vi "Angle_3.vi"() -> ()   [LabVIEW 2020]
uses:
  Support/Controls/Cmd_Mouse Popup.ctl
  Support/Controls/Clst_Initialize Input.ctl
  Support/Controls/Clst_Result inspec.ctl
  Support/Controls/Cmd_Var Data IO.ctl
  Variables/Global_Cal Info.vi
panel:
  in  "반지름":string="150" caption="투영면 반지름 (mm)"
  out "최소범위":string
  in  "표시방식":string(combo)
  out "단위":string
  out "최대범위":string
  in  "Spec 변경":bool
  in  "Random":bool
  out "Resolution":string[][](table) caption="Spec"
  out "Spec":string[][](table)
  out "제목":string
  out "에러 출력":errorcluster
  out "Condition":string[][](table) caption="2. 직선성 시험"
  in  "최소눈금":string(combo)
  in  "Measured":string[][](table) caption="투영면의 회전 각도 측정오차"
  out "Load?":bool
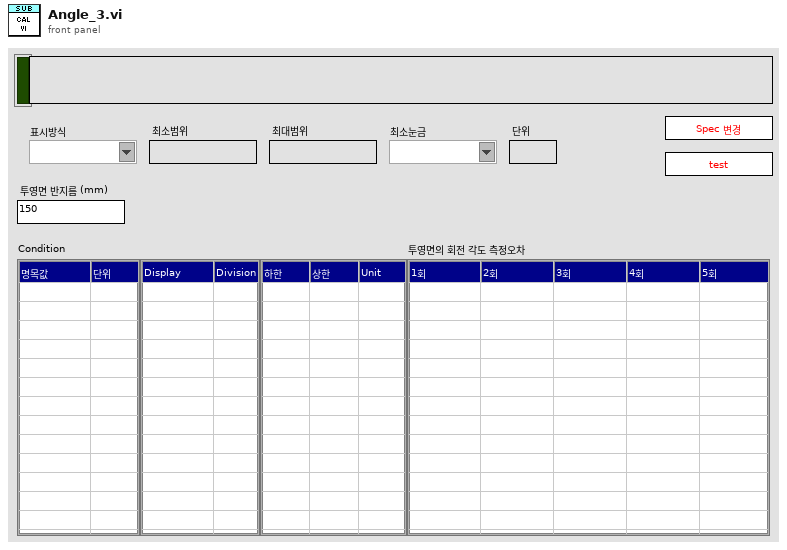
[diagram p1: front panel]
types:
  T1 = typedef "Cmd_Mouse Popup.ctl" = enum16{"활성화", "메뉴선택"}
  T2 = cluster{"Shift":bool, "Ctrl":bool, "Alt":bool, "Cmd":bool, "Opt":bool}
  T3 = typedef "Clst_Initialize Input.ctl" = cluster{"Initialize 1":cluster{"Condition":refnum<vi>[], "Spec":refnum<vi>[], "Measured":refnum<vi>[], "Resolution":refnum<vi>[], "Func_ext":string, "제목":refnum<vi>, "Measured_ADJ":refnum<vi>[]}, "Initialize 2":cluster{"문자열":refnum<vi>[], "콤보박스":refnum<vi>[], "링":refnum<vi>[], "열거형":refnum<vi>[], "테이블":refnum<vi>[], "여러열":refnum<vi>[], "디지털(DBL)":refnum<vi>[], "3D string":refnum<vi>[], "ctrl":refnum<vi>[], "boolean":refnum<vi>[]}}
  T4 = typedef "Clst_Result inspec.ctl" = cluster{"분해능":string, "문자열 1":string, "문자열 2":string, "숫자형 1":i32, "숫자형 2":i32, "숫자형 3":dbl, "문자배열 1D":string[], "문자배열 2D":string[][], "문자배열 3D":string[][][], "문자배열 4D":string[][][][], "불리언 1D":bool[]}
  T5 = typedef "Cmd_Var Data IO.ctl" = enum16{"Condition", "Condition Default", "Condition_Temp", "Resolution", "Resolution Default", "Resolution Old", "Spec", "Spec Default", "Spec Old", "Spec Temp", "Result", "Result2", "Result3", "Result_Temp", "Result_ADJ", "Result_ADJ2", "STD1", "STD2", "STD3", "STD4", "STD5", "STD Temp", "CMC", "CMC Default"}
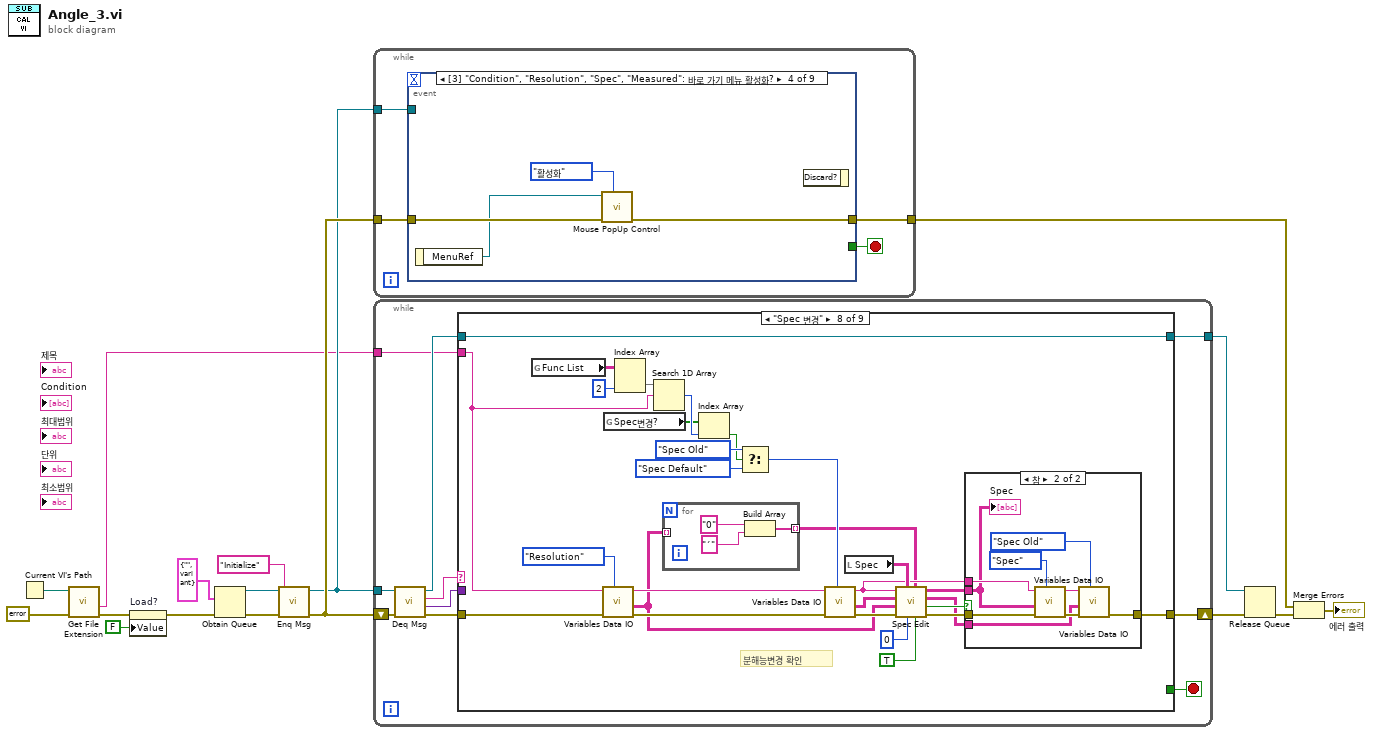
[diagram p0: block diagram]
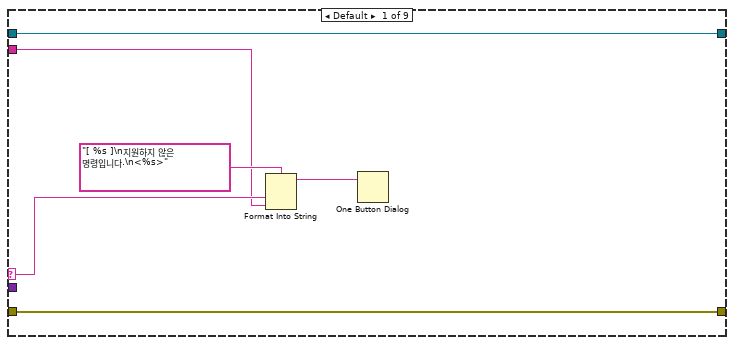
[diagram p2: hidden frame]
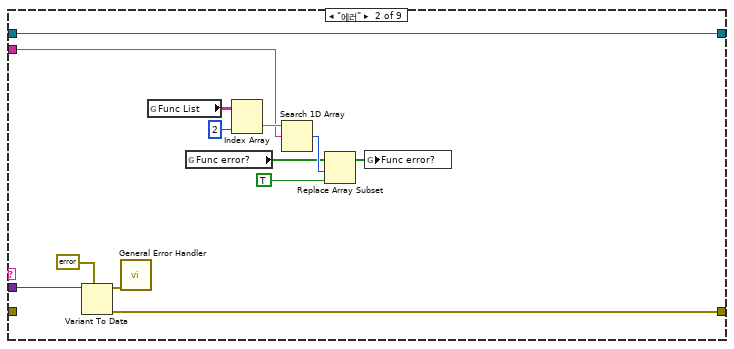
[diagram p3: hidden frame]
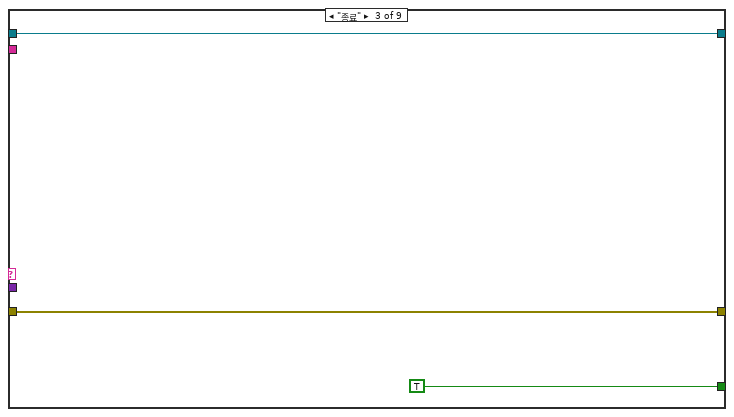
[diagram p4: hidden frame]
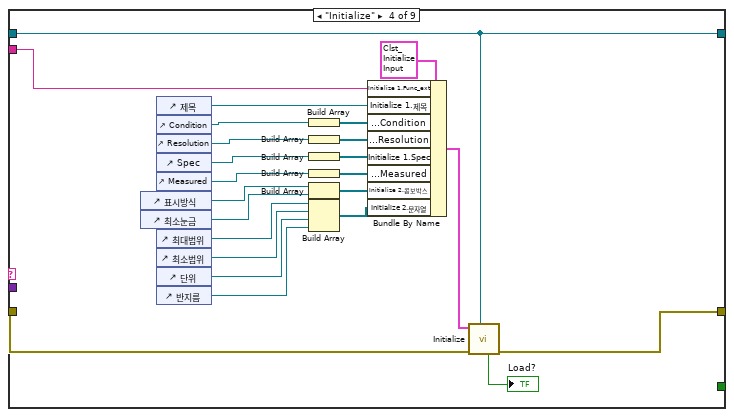
[diagram p5: hidden frame]
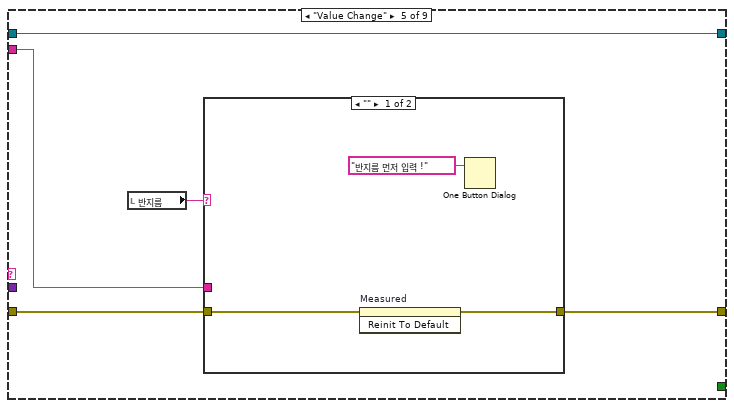
[diagram p6: hidden frame]
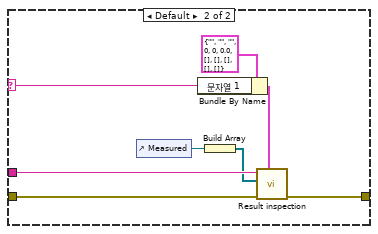
[diagram p7: hidden frame]
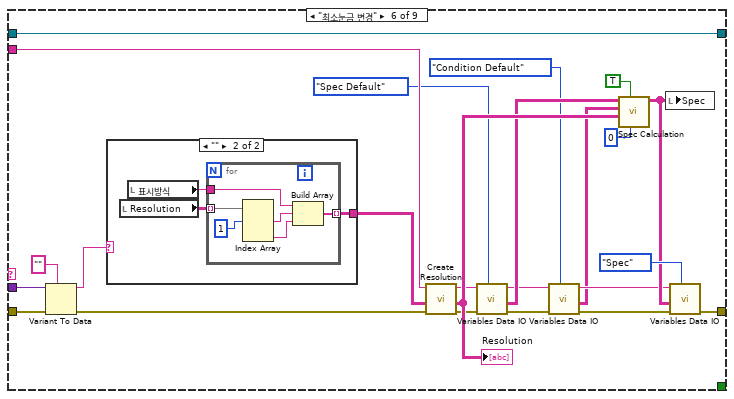
[diagram p8: hidden frame]
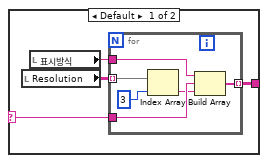
[diagram p9: hidden frame]
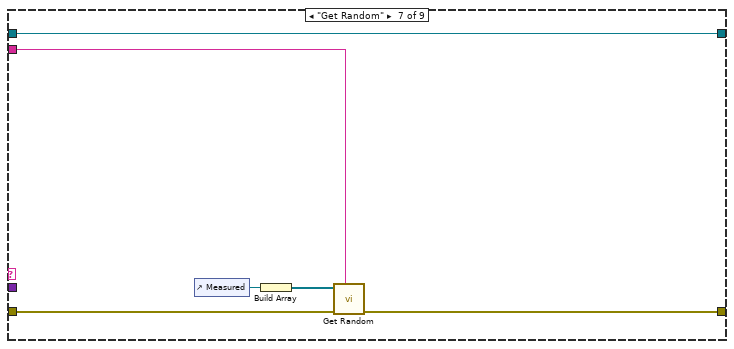
[diagram p10: hidden frame]
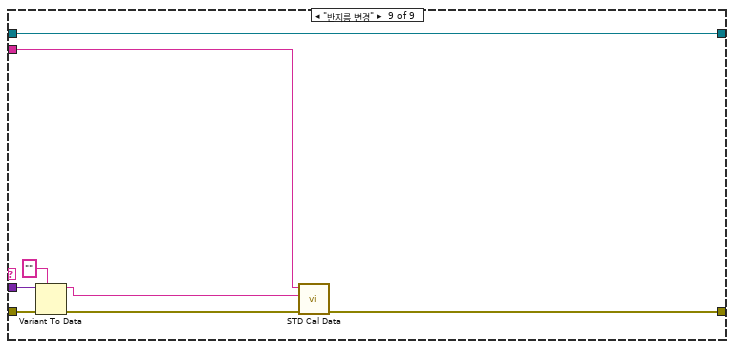
[diagram p12: hidden frame]
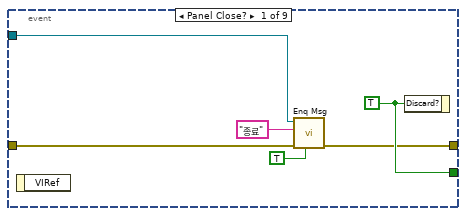
[diagram p13: hidden frame]
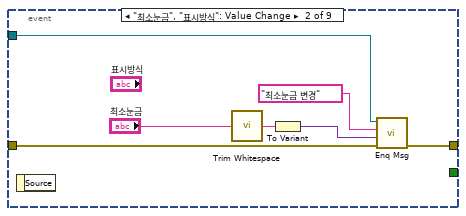
[diagram p14: hidden frame]
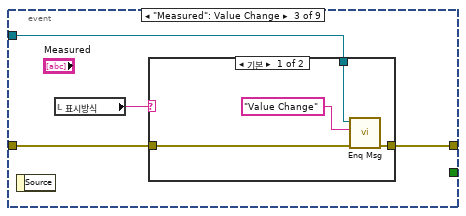
[diagram p15: hidden frame]
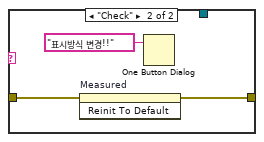
[diagram p16: hidden frame]
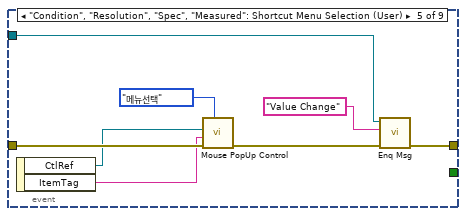
[diagram p17: hidden frame]
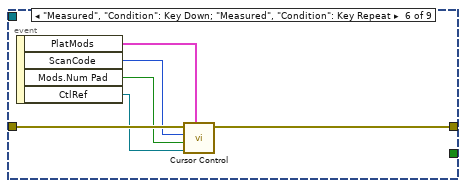
[diagram p18: hidden frame]
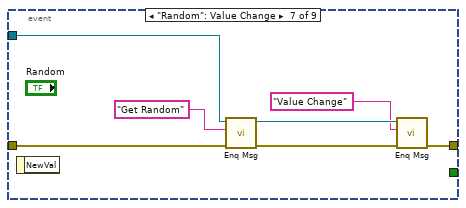
[diagram p19: hidden frame]
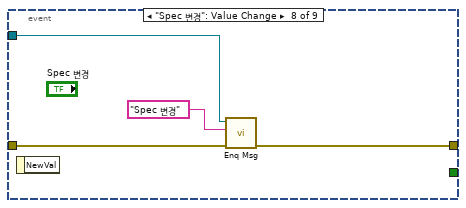
[diagram p20: hidden frame]
diagram:
  n1 = Current VI's Path() -> (path=w5:path)
  n2 = call <vilib>:"Get File Extension.vi"("error in (no error)"=errorcluster {"status"=FALSE, "code"=0, "source"=""} ("에러 상수"), "file"=w5) -> ("error out"=w3:errorcluster, "filename without extension"=w4:string)  [unwired: 5 in, 3 out]
  n3 = property on="Load?" class="Bool (엄격한)"(error in=w3, "Value"=FALSE ("Load?")) -> (error out=w2:errorcluster)  [unwired: 1 in, 1 out]
  n4 = Obtain Queue(element data type=cluster{"메세지":string, "값":variant} {"메세지"="", "값"=variant} ("Message Cluster"), error in (no error)=w2) -> (queue out=w14:refnum<queue>, error out=w16:errorcluster)  [unwired: 3 in, 1 out]
  n5 = call "Enq Msg.vi"("에러 입력(에러 없음)"=w16, "메세지"="Initialize", "큐 입력"=w14) -> ("에러 출력"=w15:errorcluster, "큐 출력"=w12:refnum<queue>)  [unwired: 7 in]
  n6 = while {
    tunnel: w15 -> [w19]
    tunnel: w12 -> [w20]
    tunnel: [w18] -> w9
    stop <- w21 stop-if-true
    n7 = event shown="[3] \"Condition\", \"Resolution\", \"Spec\", \"Measured\": 바로 가기 메뉴 활성화?" {
      selector: _ -> [_ _ _ _ _ _ _ _ _]
      dyn-events: _ -> [_ _ _ _ _ _ _ _ _]
      timeout: _ -> [_ _ _ _ _ _ _ _ _]
      tunnel: [w27 _ _ _ _ _ _ _ _] -> w21
      tunnel: w20 -> [w25 w33 w38 _ w50 _ w68 w72 w75]
      tunnel: w19 -> [w26 w34 w36 w49 w57 w63 w69 w73 w79]
      tunnel: [w23 w32 w37 w48 w51 w62 w64 w71 w78] -> w18
      event Panel Close? {
        w27 = TRUE ("버림?")
        n8 = event-data() -> ()  [unwired: 1 in, 1 out]
        n9 = call "Enq Msg.vi"("우선순위 메시지?"=TRUE, "에러 입력(에러 없음)"=w26, "메세지"="종료", "큐 입력"=w25) -> ("에러 출력"=w23:errorcluster)  [unwired: 6 in, 1 out]
        n10 = event-data("Discard?"=w27) -> ()  [unwired: 1 in, 1 out]
      }
      event "최소눈금", "표시방식": Value Change {
        n11 = event-data() -> ()  [unwired: 1 in, 1 out]
        n12 = call <vilib>:"Trim Whitespace.vi"("string"="최소눈금") -> ("trimmed string"=w30:string)  [unwired: 1 in]
        n13 = To Variant(anything=w30) -> (Variant=w28:variant)
        n14 = call "Enq Msg.vi"("에러 입력(에러 없음)"=w34, "값"=w28, "메세지"="최소눈금 변경", "큐 입력"=w33) -> ("에러 출력"=w32:errorcluster)  [unwired: 6 in, 1 out]
      }
      event "Measured": Value Change {
        n15 = event-data() -> ()  [unwired: 1 in, 1 out]
        n16 = local read "표시방식"() -> (w35:string)
        n17 = case shown="기본" w35 {
          tunnel: w38 -> [w42 _]
          tunnel: [w41 w43] -> w37
          tunnel: w36 -> [w40 w44]
          frame Default {
            n18 = call "Enq Msg.vi"("에러 입력(에러 없음)"=w40, "메세지"="Value Change", "큐 입력"=w42) -> ("에러 출력"=w41:errorcluster)  [unwired: 7 in, 1 out]
          }
          frame "Check" {
            n19 = invoke on="Measured" class="Tbl (엄격한)" method="Reinit To Default"(error in=w44) -> (error out=w43:errorcluster)  [unwired: 2 in, 2 out]
            n20 = One Button Dialog(message="표시방식 변경!!" ("메시지")) -> ()  [unwired: 1 in, 1 out]
          }
        }
      }
      event "Condition", "Resolution", "Spec", "Measured": Shortcut Menu Activation? {
        n21 = event-data() -> ("MenuRef"=w47:refnum<k9>)  [unwired: 1 in]
        n22 = call "Mouse PopUp Control.vi"("type"=Cmd_Mouse_Popup."활성화", "error in"=w49, "메뉴 참조"=w47) -> ("error out"=w48:errorcluster)  [unwired: 8 in]
        n23 = event-data() -> ()  [unwired: 2 in, 1 out]
      }
      event "Condition", "Resolution", "Spec", "Measured": Shortcut Menu Selection (User) {
        n24 = event-data() -> ("CtlRef"=w55:refnum<vi>, "ItemTag"=w54:string)  [unwired: 1 in]
        n25 = call "Mouse PopUp Control.vi"("type"=Cmd_Mouse_Popup."메뉴선택", "error in"=w57, "아이템 태그"=w54, "Tbl 참조 번호"=w55) -> ("error out"=w52:errorcluster)  [unwired: 7 in]
        n26 = call "Enq Msg.vi"("에러 입력(에러 없음)"=w52, "메세지"="Value Change", "큐 입력"=w50) -> ("에러 출력"=w51:errorcluster)  [unwired: 7 in, 1 out]
      }
      event "Measured", "Condition": Key Down; "Measured", "Condition": Key Repeat {
        n27 = event-data() -> ("PlatMods"=w58:T2, "ScanCode"=w61:i16, "Mods.Num Pad"=w60:bool, "CtlRef"=w59:refnum<vi>)  [unwired: 1 in]
        n28 = call "Cursor Control.vi"("플랫폼 조합키"=w58, "참조"=w59, "Num Pad"=w60, "ScanCode"=w61, "error in"=w63) -> ("error out"=w62:errorcluster)  [unwired: 5 in, 1 out]
      }
      event "Random": Value Change {
        n29 = event-data() -> ()  [unwired: 1 in, 1 out]
        n30 = call "Enq Msg.vi"("에러 입력(에러 없음)"=w69, "메세지"="Get Random", "큐 입력"=w68) -> ("에러 출력"=w67:errorcluster, "큐 출력"=w66:refnum<queue>)  [unwired: 7 in]
        n31 = call "Enq Msg.vi"("에러 입력(에러 없음)"=w67, "메세지"="Value Change", "큐 입력"=w66) -> ("에러 출력"=w64:errorcluster)  [unwired: 7 in, 1 out]
      }
      event "Spec 변경": Value Change {
        n32 = event-data() -> ()  [unwired: 1 in, 1 out]
        n33 = call "Enq Msg.vi"("에러 입력(에러 없음)"=w73, "메세지"="Spec 변경", "큐 입력"=w72) -> ("에러 출력"=w71:errorcluster)  [unwired: 7 in, 1 out]
      }
      event "반지름": Value Change {
        n34 = event-data() -> ()  [unwired: 1 in, 2 out]
        n35 = To Variant(anything="반지름") -> (Variant=w76:variant)
        n36 = call "Enq Msg.vi"("에러 입력(에러 없음)"=w79, "값"=w76, "메세지"="반지름 변경", "큐 입력"=w75) -> ("에러 출력"=w78:errorcluster)  [unwired: 6 in, 1 out]
      }
    }
  }
  n37 = while {
    shift-right: [w90] -> w11
    shift-left: w15 -> [w89]
    tunnel: w12 -> [w87]
    tunnel: [w82] -> w10
    tunnel: w4 -> [w81]
    stop <- w83 stop-if-true
    n38 = call "Deq Msg.vi"("에러 입력(에러 없음)"=w89, "큐 입력"=w87) -> ("에러 출력"=w88:errorcluster, "값"=w84:variant, "메세지"=w86:string, "큐 출력"=w85:refnum<queue>)  [unwired: 6 in]
    n39 = case shown="\"Spec 변경\"" w86 {
      selector: w86 -> [w92 _ _ _ _ _ _ _ _]
      tunnel: w88 -> [w96 _ w112 w136 w138 w175 w197 w222 w249]
      tunnel: [w96 w106 w112 w116 w140 w168 w198 w225 w243] -> w90
      tunnel: w85 -> [w95 w105 w110 w121 w141 w176 w201 w229 w250]
      tunnel: w84 -> [_ w107 _ _ _ w174 _ _ w247]
      tunnel: [_ _ TRUE ("버림?") _ _ _ _ _ _] -> w83
      tunnel: [w95 w105 w110 w121 w141 w176 w201 w229 w250] -> w82
      tunnel: w81 -> [w91 w97 _ w122 w139 w172 w196 w208 w244]
      frame Default {
        n40 = Format Into String(format string="[ %s ]\n지원하지 않은 명령입니다.\n<%s>" ("메시지"), w92, w91) -> (resulting string=w93:string)  [unwired: 2 in, 1 out]
        n41 = One Button Dialog(message=w93) -> ()  [unwired: 1 in, 1 out]
      }
      frame "에러" {
        n42 = Variant To Data(type=errorcluster {"status"=FALSE, "code"=0, "source"=""} ("에러 출력"), Variant=w107) -> (data=w109:errorcluster, error out=w106:errorcluster)  [unwired: 1 in]
        n43 = call <vilib>:"General Error Handler.vi"("error in (no error)"=w109) -> ()  [unwired: 10 in, 5 out]
        n44 = global read "Global_Cal Info.vi" "Func List"() -> (w99:string[][])
        n45 = global read "Global_Cal Info.vi" "Func error?"() -> (w102:bool[])
        n46 = Index Array(array=w99, index (col)=2 ("비활성화된 인덱스 (열)")) -> (element=w100:string[])  [unwired: 1 in]
        n47 = Search 1D Array(1D array=w100, element=w97) -> (index of element=w103:i32)  [unwired: 1 in]
        n48 = Replace Array Subset(array=w102, new element=TRUE ("새 원소/부분배열"), index=w103) -> (w104:bool[])
        n49 = global write "Global_Cal Info.vi" "Func error?"(w104) -> ()
      }
      frame "종료" {
      }
      frame "Initialize" {
        n50 = control-ref of="표시방식"() -> (w120:refnum<vi>)
        n51 = control-ref of="최소눈금"() -> (w129:refnum<vi>)
        n52 = control-ref of="제목"() -> (w127:refnum<vi>)
        n53 = control-ref of="Condition"() -> (w133:refnum<vi>)
        n54 = control-ref of="Resolution"() -> (w123:refnum<vi>)
        n55 = control-ref of="Spec"() -> (w126:refnum<vi>)
        n56 = control-ref of="Measured"() -> (w130:refnum<vi>)
        n57 = control-ref of="최대범위"() -> (w115:refnum<vi>)
        n58 = control-ref of="최소범위"() -> (w117:refnum<vi>)
        n59 = control-ref of="단위"() -> (w119:refnum<vi>)
        n60 = control-ref of="반지름"() -> (w113:refnum<vi>)
        n61 = Build Array(w133) -> (w132:refnum<vi>[])
        n62 = Build Array(w123) -> (w124:refnum<vi>[])
        n63 = Build Array(w126) -> (w125:refnum<vi>[])
        n64 = Build Array(w130) -> (w131:refnum<vi>[])
        n65 = Build Array(w120, w129) -> (w128:refnum<vi>[])
        n66 = Build Array(w115, w117, w119, w113) -> (w118:refnum<vi>[])
        n67 = Bundle By Name(cluster=T3 {"Initialize 1"={"Condition"=[], "Spec"=[], "Measured"=[], "Resolution"=[], "Func_ext"="", "제목"=refnum, "Measured_ADJ"=[]}, "Initialize 2"={"문자열"=[], "콤보박스"=[], "링"=[], "열거형"=[], "테이블"=[], "여러열"=[], "디지털(DBL)"=[], "3D string"=[], "ctrl"=[], "boolean"=[]}} ("입력 클러스터"), "Initialize 1.Func_ext"=w122, "Initialize 1.제목"=w127, "Initialize 1.Condition"=w132, "Initialize 1.Resolution"=w124, "Initialize 1.Spec"=w125, "Initialize 1.Measured"=w131, "Initialize 2.콤보박스"=w128, "Initialize 2.문자열"=w118) -> (w134:T3)
        n68 = call "Initialize.vi"("큐 입력"=w121, "error in"=w136, "입력 클러스터"=w134) -> ("error out"=w116:errorcluster, "Load?"=→"Load?":bool)  [unwired: 5 in, 2 out]
      }
      frame "Value Change" {
        n69 = local read "반지름"() -> (w137:string)
        n70 = case shown="\"\"" w137 {
          selector: w137 -> [_ w145]
          tunnel: [w143 w152] -> w140
          tunnel: w139 -> [_ w151]
          tunnel: w138 -> [w144 w150]
          frame "" {
            n71 = invoke on="Measured" class="Tbl (엄격한)" method="Reinit To Default"(error in=w144) -> (error out=w143:errorcluster)  [unwired: 2 in, 2 out]
            n72 = One Button Dialog(message="반지름 먼저 입력 !" ("메시지")) -> ()  [unwired: 1 in, 1 out]
          }
          frame Default {
            n73 = control-ref of="Measured"() -> (w149:refnum<vi>)
            n74 = Bundle By Name(cluster=T4 {"분해능"="", "문자열 1"="", "문자열 2"="", "숫자형 1"=0, "숫자형 2"=0, "숫자형 3"=0.0, "문자배열 1D"=[], "문자배열 2D"=[], "문자배열 3D"=[], "문자배열 4D"=[], "불리언 1D"=[]} ("입력 클러스터"), "문자열 1"=w145) -> (w146:T4)
            n75 = Build Array(w149) -> (w148:refnum<vi>[])
            n76 = call "Result inspection.vi"("입력 클러스터"=w146, "error in"=w150, "Ref. Data (Inspection)"=w148, "Func ext"=w151) -> ("error out"=w152:errorcluster)  [unwired: 4 in, 3 out]
          }
        }
      }
      frame "최소눈금 변경" {
        n77 = Variant To Data(error in=w175, type="", Variant=w174) -> (data=w161:string, error out=w163:errorcluster)
        n78 = case shown="\"\"" w161 {
          selector: w161 -> [w177 _]
          tunnel: [w180 w189] -> w162
          frame Default {
            n79 = local read "Resolution"() -> (w179:string[][])
            n80 = local read "표시방식"() -> (w178:string)
            n81 = for {
              tunnel: w179 -> [w186] mode=indexing
              tunnel: w177 -> [w185]
              tunnel: [w183] -> w180 mode=indexing
              tunnel: w178 -> [w182]
              n82 = Index Array(array=w186, index=3 ("인덱스")) -> (element=w184:string)
              n83 = Build Array(w182, w185, w184) -> (w183:string[])
            }
          }
          frame "" {
            n84 = local read "Resolution"() -> (w188:string[][])
            n85 = local read "표시방식"() -> (w187:string)
            n86 = for {
              tunnel: w188 -> [w195] mode=indexing
              tunnel: [w194] -> w189 mode=indexing
              tunnel: w187 -> [w193]
              n87 = Index Array(array=w195, index #1=1 ("인덱스")) -> (element #1=w191:string, element #3=w190:string)  [unwired: 2 in, 1 out]
              n88 = Build Array(w193, w191, w190) -> (w194:string[])
            }
          }
        }
        n89 = call "Create Resolution.vi"("에러 입력(에러 없음)"=w163, "Resolution"=w162, "Func_ext"=w172) -> ("에러 출력"=w166:errorcluster, "Resolution Out"=w169:string[][], "Func_ext 출력"=w165:string)  [unwired: 6 in]
        "Resolution" <- w169
        n90 = call "Variables Data IO.vi"("Select"=Cmd_Var_Data_IO."Spec Default", "error in"=w166, "Func_ext"=w165) -> ("error out"=w157:errorcluster, "Data Out"=w164:string[][], "Func_ext Out"=w158:string)  [unwired: 6 in]
        n91 = call "Variables Data IO.vi"("Select"=Cmd_Var_Data_IO."Condition Default", "error in"=w157, "Func_ext"=w158) -> ("error out"=w155:errorcluster, "Data Out"=w154:string[][], "Func_ext Out"=w156:string)  [unwired: 6 in]
        n92 = call "Spec Calculation.vi"("기준값 열번호"=0 ("열번호(기준값)"), "0기준?"=TRUE, "Resolution"=w169, "Condition in"=w154, "Spec Default"=w164) -> ("Spec out"=w160:string[][])  [unwired: 5 in, 1 out]
        n93 = local write "Spec"(w160) -> ()
        n94 = call "Variables Data IO.vi"("Select"=Cmd_Var_Data_IO."Spec", "error in"=w155, "Data In"=w160, "Func_ext"=w156) -> ("error out"=w168:errorcluster)  [unwired: 5 in, 2 out]
      }
      frame "Get Random" {
        n95 = control-ref of="Measured"() -> (w200:refnum<vi>)
        n96 = Build Array(w200) -> (w199:refnum<vi>[])
        n97 = call "Get Random.vi"("Func_Ext"=w196, "에러 입력"=w197, "Meas"=w199) -> ("에러 출력"=w198:errorcluster)  [unwired: 7 in, 1 out]
      }
      frame "Spec 변경" {
        # "분해능변경 확인"
        n98 = global read "Global_Cal Info.vi" "Func List"() -> (w213:string[][])
        n99 = call "Variables Data IO.vi"("Select"=Cmd_Var_Data_IO."Resolution", "error in"=w222, "Func_ext"=w208) -> ("error out"=w206:errorcluster, "Data Out"=w204:string[][], "Func_ext Out"=w205:string)  [unwired: 6 in]
        n100 = global read "Global_Cal Info.vi" "Spec변경?"() -> (w209:bool[])
        n101 = Index Array(array=w213, index (col)=2 ("비활성화된 인덱스 (열)")) -> (element=w211:string[])  [unwired: 1 in]
        n102 = Search 1D Array(1D array=w211, element=w208) -> (index of element=w210:i32)  [unwired: 1 in]
        n103 = for {
          tunnel: w204 -> [_] mode=indexing
          tunnel: [w230] -> w203 mode=indexing
          n104 = Build Array("0" ("원소"), "´" ("원소")) -> (w230:string[])
        }
        n105 = Index Array(array=w209, index=w210) -> (element=w214:bool)
        n106 = Select(t=Cmd_Var_Data_IO."Spec Old" ("Select"), s=w214, f=Cmd_Var_Data_IO."Spec Default" ("Select")) -> (s? t:f=w207:T5)
        n107 = call "Variables Data IO.vi"("Select"=w207, "error in"=w206, "Func_ext"=w205) -> ("error out"=w224:errorcluster, "Data Out"=w217:string[][], "Func_ext Out"=w218:string)  [unwired: 6 in]
        n108 = local read "Spec"() -> (w219:string[][])
        n109 = call "Spec Edit.vi"("0기준?"=TRUE, "Condition"=w203, "열번호(기준값)"=0, "Spec Value"=w219, "에러 입력(에러 없음)"=w224, "Resolution"=w204, "Spec Default"=w217, "Func_ext"=w218) -> ("에러 출력"=w226:errorcluster, "변경?"=w227:bool, "Spec Default out"=w221:string[][], "Spec 출력"=w228:string[][])
        n110 = case shown="참" w227 {
          tunnel: w228 -> [_ w239]
          tunnel: w226 -> [w233 w242]
          tunnel: [w233 w237] -> w225
          tunnel: w218 -> [_ w240]
          tunnel: w221 -> [_ w235]
          frame False {
          }
          frame True {
            n111 = call "Variables Data IO.vi"("Select"=Cmd_Var_Data_IO."Spec", "error in"=w242, "Data In"=w239, "Func_ext"=w240) -> ("error out"=w238:errorcluster, "Func_ext Out"=w236:string)  [unwired: 5 in, 1 out]
            n112 = call "Variables Data IO.vi"("Select"=Cmd_Var_Data_IO."Spec Old", "error in"=w238, "Data In"=w235, "Func_ext"=w236) -> ("error out"=w237:errorcluster)  [unwired: 5 in, 2 out]
            "Spec" <- w239
          }
        }
      }
      frame "반지름 변경" {
        n113 = Variant To Data(error in=w249, type="", Variant=w247) -> (data=w245:string, error out=w248:errorcluster)
        n114 = call "STD Cal Data.vi"("error in"=w248, "문자열"=w245, "Func_ext"=w244) -> ("error out"=w243:errorcluster)  [unwired: 4 in, 4 out]
      }
    }
  }
  n115 = Release Queue(queue=w10, error in (no error)=w11) -> (error out=w8:errorcluster)  [unwired: 1 in, 2 out]
  n116 = Merge Errors(w9, w8) -> (→"에러 출력":errorcluster)
